vi "Add Prompt.vi"(8 "error in (no error)":errorcluster, 10 "vi path":path, 11 "server id":i32) -> (0 "error out":errorcluster, 3 "server id out":i32)   [LabVIEW 2020, in "MCP Server.lvlib"]
doc: "Adds a prompt to the MCP server. The prompt callback VIs string input controls on the connector pane will be used as arguments. To add a description to an argument, add a description to the controls properties. The name and description of the VI will be used as name and description for the prompt.S"
uses:
  MCP Server.lvlib
  Prompt Data.ctl
  Prompt Argument.ctl
  <vilib>/Utility/error.llb/Error Cluster From Error Code.vi
  <vilib>/ErrorRing/Error Ring.xnode
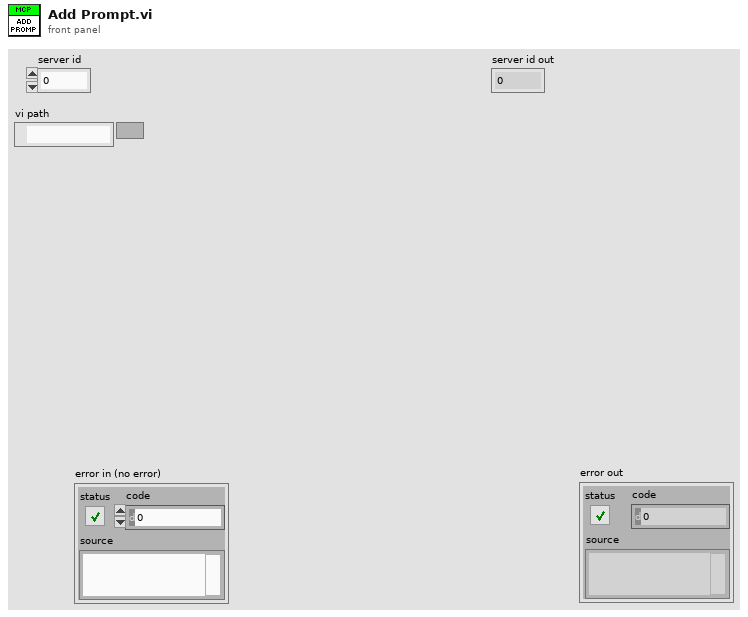
[diagram p1: front panel]
types:
  T1 = typedef "MCP Server.lvlib/Prompt Data.ctl" = cluster{"name":string, "description":string, "arguments":T2[], "return terminal name":string, "results description":string, "VI Refnum":refnum<vi>}
  T2 = typedef "MCP Server.lvlib/Prompt Argument.ctl" = cluster{"name":string, "description":string, "required":bool, "raw_name":string}
  T3 = typedef "MCP Server.lvlib/Terminal.ctl" = cluster{"Name":string, "Type":string, "IsIndicator?":bool, "IsRequired?":bool, "Description":string, "sub type":string, "array dimensions":i32}
  T4 = typedef "MCP Server.lvlib/Server Data.ctl" = cluster{"Name":string, "Description":string, "Tools":T5[], "Parameters":string[][], "Logging Info":T8, "User Events":T9, "Prompts":T1[], "resources":T10[], "HTTP Server":refnum<class "Server.lvclass">}
  T5 = typedef "MCP Server.lvlib/Tool Data.ctl" = cluster{"Name":string, "Description":string, "Ignored":string[], "inputs":T6[], "outputs":T7[], "VI Refnum":refnum<vi>}
  T6 = typedef "MCP Server.lvlib/Input Parameter.ctl" = cluster{"name":string, "type":string, "description":string, "required":bool, "raw name":string}
  T7 = typedef "MCP Server.lvlib/Output Parameter.ctl" = cluster{"name":string, "description":string, "type":string, "raw name":string}
  T8 = typedef "MCP Server.lvlib/Logging.ctl" = cluster{"Log":string[], "Max Length":i32}
  T9 = typedef "MCP Server.lvlib/User Events.ctl" = cluster{"onError":refnum<user-event>, "onRpc":refnum<user-event>}
  T10 = typedef "MCP Server.lvlib/resource data.ctl" = cluster{"uri":string, "name":string, "description":string, "mimeType":string, "file path":path}
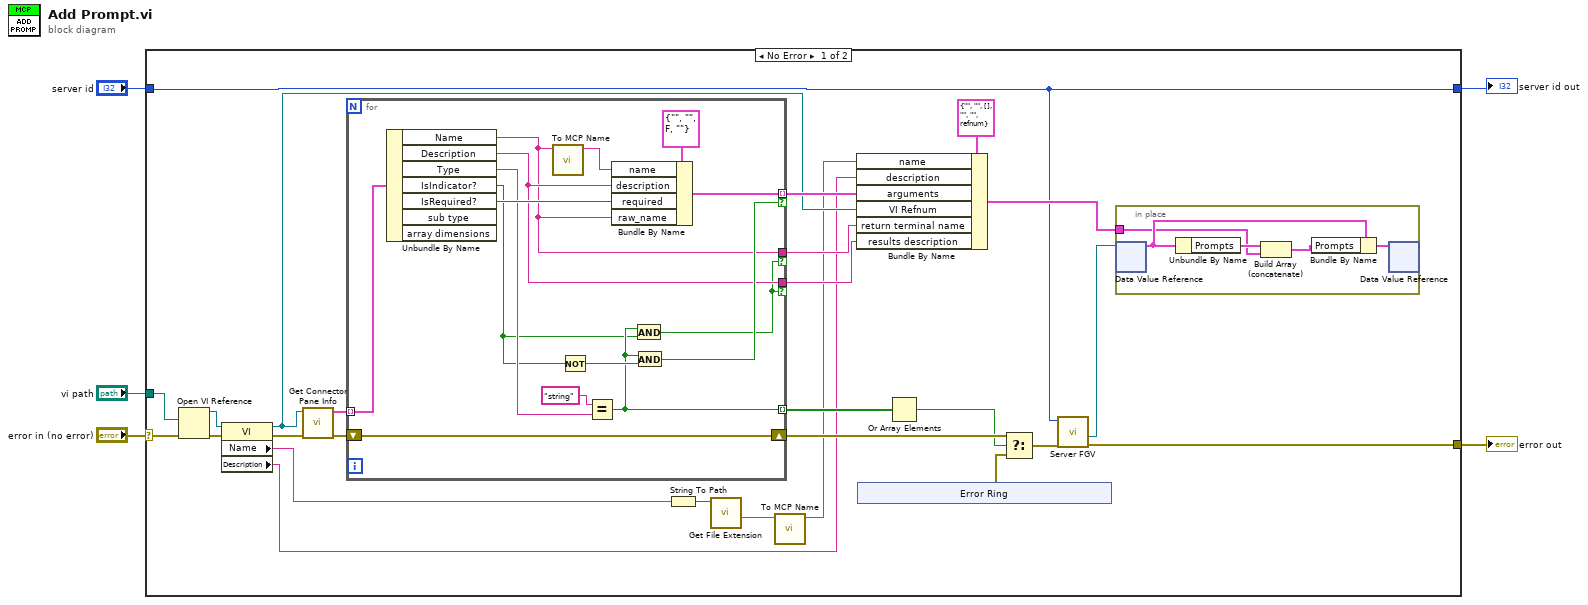
[diagram p0: block diagram]
diagram:
  n1 = case shown="No Error" "error in (no error)" {
    selector: "error in (no error)" -> [w7 w57]
    tunnel: [w31 w57] -> w5
    tunnel: "server id" -> [w6 w58]
    tunnel: "vi path" -> [w22 _]
    tunnel: [w6 w58] -> w2
    frame No Error {
      n2 = Open VI Reference(vi path=w22, error in (no error)=w7) -> (vi reference=w14:refnum<vi>, error out=w23:errorcluster)  [unwired: 4 in]
      n3 = property class="VI"(reference=w14, error in=w23) -> (reference out=w13:refnum<vi>, error out=w15:errorcluster, "Name"=w9:string, "Description"=w12:string)
      n4 = call "Get Connector Pane Info.vi"("error in (no error)"=w15, "vi reference"=w13) -> ("error out"=w25:errorcluster, "Terminals"=w28:T3[])  [unwired: 8 in]
      n5 = for {
        tunnel: w28 -> [w51] mode=indexing
        tunnel: [w46] -> w27 mode=indexing if=w45
        shift-right: [w44] -> w24
        shift-left: w25 -> [w44]
        tunnel: [w41] -> w21 if=w38
        tunnel: [w39] -> w20 mode=indexing
        tunnel: [w42] -> w16 if=w38
        n6 = Unbundle By Name(w51) -> ("Name"=w41:string, "Description"=w42:string, "Type"=w43:string, "IsIndicator?"=w37:bool, "IsRequired?"=w47:bool)  [unwired: 2 out]
        n7 = call "To MCP Name.vi"("unformatted name"=w41) -> ("MCP name"=w40:string)  [unwired: 10 in]
        n8 = Not(x=w37) -> (.not. x?=w49:bool)
        n9 = Equal?(x="string", y=w43) -> (x = y?=w39:bool)
        n10 = Bundle By Name(cluster=T2 {"name"="", "description"="", "required"=FALSE, "raw_name"=""} ("Prompt Argument"), "name"=w40, "description"=w42, "required"=w47, "raw_name"=w41) -> (w46:T2)
        n11 = And(x=w39, y=w37) -> (x .and. y?=w38:bool)
        n12 = And(x=w39, y=w49) -> (x .and. y?=w45:bool)
      }
      n13 = String To Path(string=w9) -> (path=w11:path)
      n14 = call <vilib>:"Get File Extension.vi"("file"=w11) -> ("filename without extension"=w10:string)  [unwired: 6 in, 4 out]
      n15 = call "To MCP Name.vi"("unformatted name"=w10) -> ("MCP name"=w8:string)  [unwired: 10 in]
      n16 = Bundle By Name(cluster=T1 {"name"="", "description"="", "arguments"=[], "return terminal name"="", "results description"="", "VI Refnum"=refnum} ("Prompt Data"), "name"=w8, "description"=w12, "arguments"=w27, "VI Refnum"=w13, "return terminal name"=w21, "results description"=w16) -> (w26:T1)
      n17 = xnode "Error Ring"() -> ("error out"=w17:errorcluster)
      n18 = Or Array Elements(Boolean array=w20) -> (logical OR=w18:bool)
      n19 = Select(t=w24, s=w18, f=w17) -> (s? t:f=w19:errorcluster)
      n20 = call "Server FGV.vi"("error in"=w19, "id"=w6) -> ("error out"=w31:errorcluster, "server reference"=w30:refnum<data-value>)  [unwired: 5 in, 3 out]
      n21 = in-place {
        in-place-border: w26 -> [w52]
        n22 = in-place-dvr #1(w30) -> (w55:T4)  [unwired: 1 out]
        n23 = Unbundle By Name(w55) -> ("Prompts"=w54:T1[])
        n24 = Build Array (concatenate)(w54, w52) -> (w53:T1[])
        n25 = Bundle By Name(cluster=w55, "Prompts"=w53) -> (w56:T4)
        n26 = in-place-dvr #1(w56) -> ()  [unwired: 2 out]
      }
    }
    frame Error {
    }
  }
  "error out" <- w5
  "server id out" <- w2
